vi "setEnableSpeedCtrl_DriveQuadTalonSRX.vi"(9 "Enable Speed Control":bool) -> ()   [LabVIEW 2019, in "DriveQuadTalonSRX_Motor.lvlib"]
uses:
  DriveQuadTalonSRX_Motor.lvlib
  globals_DriveQuadTalonSRX.vi
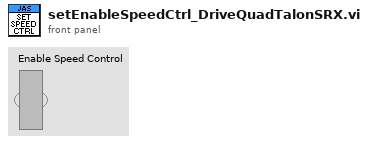
[diagram p1: front panel]
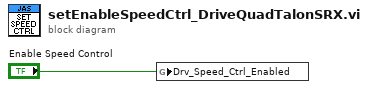
[diagram p0: block diagram]
diagram:
  n1 = global write "globals_DriveQuadTalonSRX.vi" "Drv_Speed_Ctrl_Enabled"("Enable Speed Control") -> ()
